vi "Fail.vi"(7 "Caller":string, 8 "error in (no error)":errorcluster, 9 "Message":string, 10 "Assertion":string, 11 "Caraya Test Framework in":refnum<class "Caraya Test Framework.lvclass">) -> (0 "error out":errorcluster, 3 "Caraya Test Framework out":refnum<class "Caraya Test Framework.lvclass">)   [LabVIEW 2017, in "Caraya Test Framework.lvclass"]
doc: "Executes the unit test framework-specific operation to indicate a failing test."
uses:
  Caraya Test Framework.lvclass
  Caraya Adapter/Caraya Adapter.lvclass
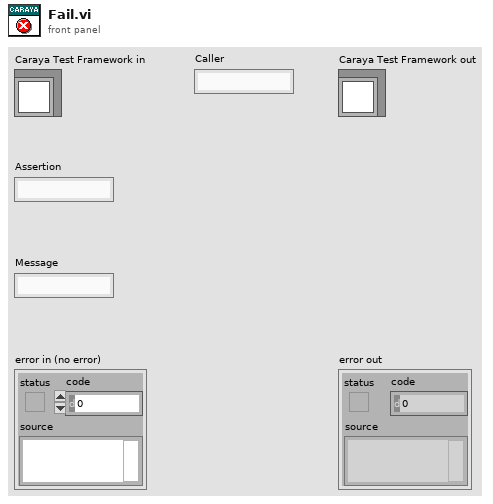
[diagram p1: front panel]
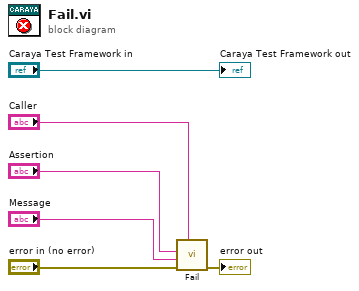
[diagram p0: block diagram]
diagram:
  n1 = call "Fail.vi"("Caller"="Caller", "error in (no error)"="error in (no error)", "Message"="Message", "Assertion"="Assertion") -> ("error out"=→"error out":errorcluster)  [unwired: 7 in]
  "Caraya Test Framework out" <- "Caraya Test Framework in"
